vi "dvp Vi Set Trigger Delay.vi"(10 "TriggerDelay":dbl, 11 "handle":u32) -> (3 "function return":u32(ring))   [LabVIEW 2018, in "LabViewDVPCamera.lvlib"]
doc: "LabviewDvp2Api dvpStatus dvpViSetTriggerDelay(dvpHandle handle, double TriggerDelay);"
uses:
  LabViewDVPCamera.lvlib
  LabViewDVPCamera/LabViewDVPCamera.dll
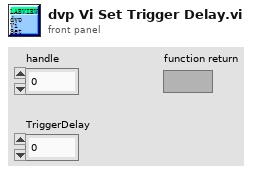
[diagram p1: front panel]
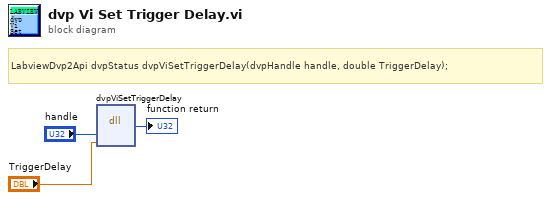
[diagram p0: block diagram]
diagram:
  # "LabviewDvp2Api dvpStatus dvpViSetTriggerDelay(dvpHandle handle, double TriggerDelay);"
  n1 = dll-call lib="C:/Program Files (x86)/DVP2 Labview cn 64/Sample/LabViewDVPCamera/LabViewDVPCamera.*" fn="dvpViSetTriggerDelay"("handle"="handle", "TriggerDelay"="TriggerDelay") -> (→"function return":u32)  [unwired: 5 in, 2 out]
